vi "InitListbox.vi"(8 "error in (no error)":errorcluster, 11 "DisplayWindow in":refnum<class "DisplayWindow.lvclass">) -> (0 "error out":errorcluster, 3 "DisplayWindow out":refnum<class "DisplayWindow.lvclass">)   [LabVIEW 2016, in "DisplayWindow.lvlib" / "DisplayWindow.lvclass"]
uses:
  DisplayWindow.lvclass
  DisplayWindow.lvclass/DisplayWindow.ctl
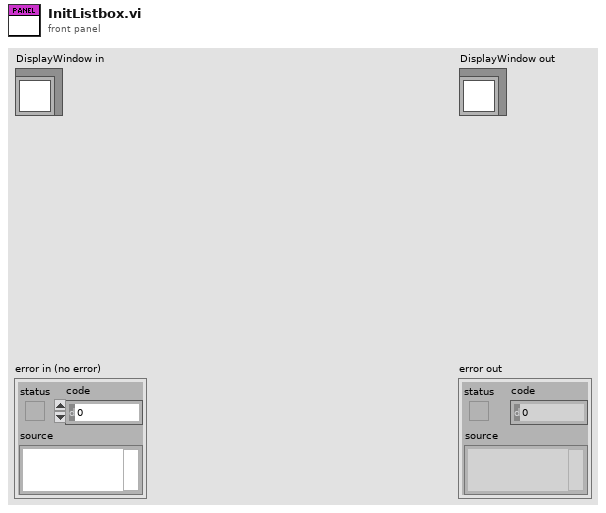
[diagram p1: front panel]
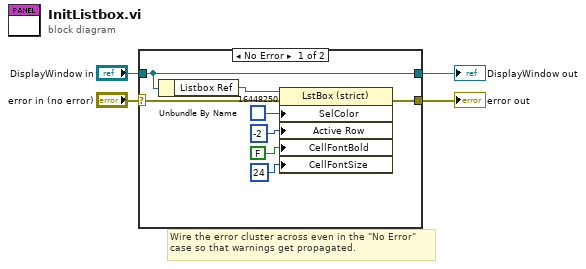
[diagram p0: block diagram]
diagram:
  # "Wire the error cluster across even in the \"No Error\"\ncase so that warnings get propagated."
  n1 = case shown="No Error" "error in (no error)" {
    selector: "error in (no error)" -> [w10 w14]
    tunnel: [w9 w14] -> w3
    tunnel: [w12 w13] -> w1
    tunnel: "DisplayWindow in" -> [w12 w13]
    frame No Error {
      n2 = Unbundle By Name(w12) -> ("Listbox Ref"=w11:refnum<vi>)
      n3 = property on="Property Node" class="LstBox (strict)"(reference=w11, error in=w10, "SelColor"=u32 16448250, "Active Row"=-2 ("Active Row:Active Row Number"), "CellFontBold"=FALSE ("Active Row:Cell Font:Bold"), "CellFontSize"=u32 24 ("Active Row:Cell Font:Size")) -> (error out=w9:errorcluster)  [unwired: 1 out]
    }
    frame Error {
    }
  }
  "error out" <- w3
  "DisplayWindow out" <- w1
